vi "Write target.vi"(8 "error in (no error)":errorcluster, 10 "Target.lvclass":refnum<class "Target.lvclass">, 11 "TargetConfiguration in":refnum<class "TargetConfiguration.lvclass">) -> (0 "error out":errorcluster, 3 "TargetConfiguration out":refnum<class "TargetConfiguration.lvclass">)   [LabVIEW 2014, in "TCSDataDefinitions.lvlib" / "TCSCommand.lvlib" / "TargetConfiguration.lvlib" / "TargetConfiguration.lvclass"]
uses:
  TargetConfiguration.lvclass
  Target/Target/Target.lvclass
  TargetConfiguration.lvclass/TargetConfiguration.ctl
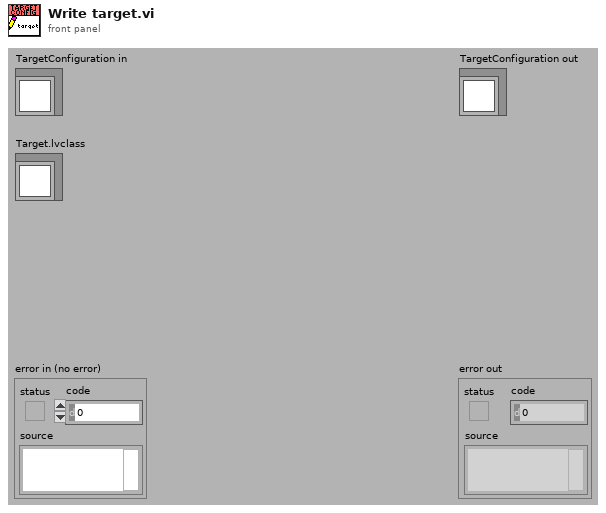
[diagram p1: front panel]
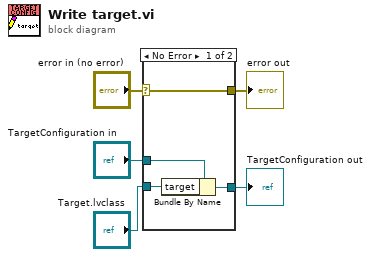
[diagram p0: block diagram]
diagram:
  n1 = case shown="No Error" "error in (no error)" {
    selector: "error in (no error)" -> [w9 w10]
    tunnel: [w9 w10] -> w4
    tunnel: [w7 w11] -> w2
    tunnel: "TargetConfiguration in" -> [w8 w11]
    tunnel: "Target.lvclass" -> [w6 _]
    frame No Error {
      n2 = Bundle By Name(cluster=w8, "target"=w6) -> (w7:refnum<class "TargetConfiguration.lvclass">)
    }
    frame Error {
    }
  }
  "error out" <- w4
  "TargetConfiguration out" <- w2
